vi "niFPGA BFGroup Twiddle Table 2048 U32 Inv.vi"(7 "address":fxp<+,11,11>) -> (4 "twid real":fxp<+/-,17,2> format="%.16g", 6 "twid imag":fxp<+/-,17,2> format="%.16g")   [LabVIEW 2017]
uses:
  <vilib>/Utility/error.llb/Clear Errors.vi
  <vilib>/rvi/Emulation/niFpgaSctlEmulationGetInTimedLoop.vi
  <vilib>/rvi/DataTransferAndStorage/Container/Common/niFpgaContainerGetUniqueNameForEmu.vi
  <vilib>/rvi/DataTransferAndStorage/Container/Common/niFpgaContainerSetEmuInfo.vi
  <vilib>/rvi/eio/common/nirviEmuReportErrorAndStop.vi
  <vilib>/rvi/Memory/Memory_Emulation/nirvimemoryEmulation.vi
  <vilib>/rvi/Memory/Memory_Emulation/nirvimemoryFastEmulation.vi
  <vilib>/rvi/Memory/Memory_Emulation/niFpgaMemoryEmulationCacheClearOnFirstRun.vi
  <vilib>/rvi/Memory/Memory_Emulation/nirvimemoryEmulationManagerCache_MakeExclusive.vi
  <vilib>/rvi/Memory/Memory_Emulation/niFpgaMemoryEmulationValidateCache.vi
  <vilib>/rvi/Memory/Memory_Emulation/nirvimemoryEmulationManagerCache_InsertValue.vi
  <vilib>/rvi/Memory/Memory_Emulation/nirvimemoryEmulationManagerCache_ReleaseExclusive.vi
  <vilib>/rvi/Memory/Memory_Emulation/nirvimemoryEmulationManagerCache_GetValue.vi
  <vilib>/rvi/Emulation/niFpgaEmulationIsFPGAContextNoSignature.vi
  <vilib>/rvi/Memory/Memory_Emulation/nirvimemoryEmulationManagerCache_SetValue.vi
  <vilib>/rvi/Emulation/niFpgaSctlEmulationResourceMgr.vi
  <vilib>/rvi/LocalResourceManager/LocalResourceManager.xnode
  <vilib>/rvi/DataTransferAndStorage/Container/XNode/niFpgaContainer.xnode
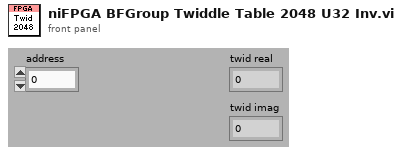
[diagram p1: front panel]
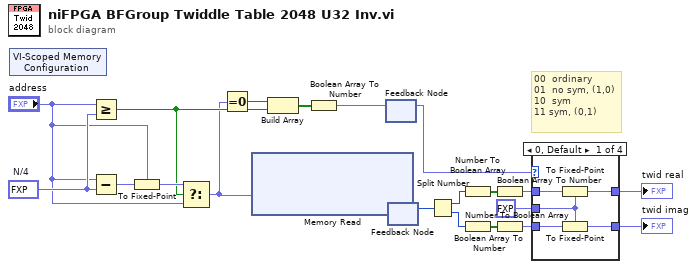
[diagram p0: block diagram]
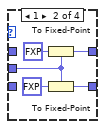
[diagram p2: hidden frame]
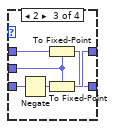
[diagram p3: hidden frame]
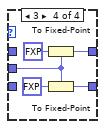
[diagram p4: hidden frame]
diagram:
  w16 = fxp<+,11,11> 1024.0  # N/4
  # "00  ordinary\n01  no sym, (1,0)\n10  sym\n11 sym, (0,1)"
  n1 = xnode "VI-Scoped Memory Configuration"() -> ()  [unwired: 1 out]
  n2 = Greater Or Equal?(x="address", y=w16) -> (x >= y?=w8:bool)
  n3 = Subtract(x="address", y=w16) -> (x-y=w15:fxp<+/-,12,12>)
  n4 = To Fixed-Point(fixed-point type="address", number=w15) -> (fixed-point=w14:fxp<+,11,11>)
  n5 = Select(t=w14, s=w8, f="address") -> (s? t:f=w2:fxp<+,11,11>)
  n6 = Equal To 0?(x=w2) -> (x = 0?=w6:bool)
  n7 = xnode ("Memory Read")("Address"=w2) -> ("Data"=w1:u32)  [unwired: 2 out]
  n8 = Build Array(w6, w8) -> (w9:bool[])
  n9 = Boolean Array To Number(Boolean array=w9) -> (number=w7:fxp<+,2,2>)
  n10 = feedback-in #1(w7) -> ()
  n11 = feedback #1() -> (w12:fxp<+,2,2>)  [unwired: 1 out]
  n12 = feedback-in #2(w1) -> ()
  n13 = feedback #2() -> (w17:u32)  [unwired: 1 out]
  n14 = Split Number(x=w17) -> (hi(x)=w20:u16, lo(x)=w18:u16)
  n15 = Number To Boolean Array(number=w20) -> (Boolean array=w21:bool[])
  n16 = Number To Boolean Array(number=w18) -> (Boolean array=w19:bool[])
  n17 = Boolean Array To Number(Boolean array=w21) -> (number=w11:fxp<+/-,16,1>)
  n18 = Boolean Array To Number(Boolean array=w19) -> (number=w10:fxp<+/-,16,1>)
  n19 = case shown="0, Default" w12 {
    tunnel: w11 -> [w26 _ w34 _]
    tunnel: [w25 w30 w35 w41] -> w4
    tunnel: w10 -> [w22 _ w36 _]
    tunnel: [w24 w28 w32 w39] -> w3
    tunnel: fxp<+/-,17,2> 0.0 ("fixed-point type") -> [w23 w27 w33 w38]
    frame 0, Default {
      n20 = To Fixed-Point(fixed-point type=w23, number=w26) -> (fixed-point=w25:fxp<+/-,17,2>)
      n21 = To Fixed-Point(fixed-point type=w23, number=w22) -> (fixed-point=w24:fxp<+/-,17,2>)
    }
    frame 1 {
      n22 = To Fixed-Point(fixed-point type=w27, number=fxp<+,1,1> 1.0 ("fixed-point type")) -> (fixed-point=w30:fxp<+/-,17,2>)
      n23 = To Fixed-Point(fixed-point type=w27, number=fxp<+,1,1> 0.0 ("fixed-point type")) -> (fixed-point=w28:fxp<+/-,17,2>)
    }
    frame 2 {
      n24 = Negate(x=w36) -> (-x=w37:fxp<+/-,17,2>)
      n25 = To Fixed-Point(fixed-point type=w33, number=w34) -> (fixed-point=w32:fxp<+/-,17,2>)
      n26 = To Fixed-Point(fixed-point type=w33, number=w37) -> (fixed-point=w35:fxp<+/-,17,2>)
    }
    frame 3 {
      n27 = To Fixed-Point(fixed-point type=w38, number=fxp<+,1,1> 0.0 ("fixed-point type")) -> (fixed-point=w41:fxp<+/-,17,2>)
      n28 = To Fixed-Point(fixed-point type=w38, number=fxp<+,1,1> 1.0 ("fixed-point type")) -> (fixed-point=w39:fxp<+/-,17,2>)
    }
  }
  "twid real" <- w4
  "twid imag" <- w3
